vi "Tektronix TDS 3000 Series Dual channel Waveform Acquire.vi"() -> ()   [LabVIEW 2010]
doc: "DESCRIPTION:\nThis VI shows how to configure the Tektronix TDS 3xxx Series for a dual-channel waveform acquisition. It uses edge triggering to trigger the acquisition. \n\nINSTRUCTIONS:\n1. Pass a valid VISA session\n2. Enter a vertical offset, range and coupling for the specified channels.\n3. Enter the probe attenuation for the probe attached to the specified channel inputs.\n4. Enter the acquisition start time and desired time per record you want in the record.\n5. Enter the trigger level for the edge trigger.\n6. Run the VI.\n7. The acquired waveforms will be displayed in the graph.\n\nNOTES:\nNotice the order of the Tektronix tktd3k component VIs in the block diagram.\n\nThis VI sets the following controls on the block diagram:\n 20MHz Max Input Frequency.\n 1.0M Ohm Input Impedance.\n 500ns trigger holdoff.\n Edge trigger is DC coupled with a positive slope.\nTo change these controls, modify the associated block diagram constants."
uses:
  <instrlib>/Tektronix TDS 3000 Series/Tektronix TDS 3000 Series.lvlib
panel:
  in  "Acquisition Start Time (0.0 s)":dbl format="%.2p"
  in  "Trigger Source (Chan 1)":string(combo)="CH1"
  in  "Trigger Level (1.0 V)":dbl=1.0 format="%.2p"
  in  "Time Per Record (4.0e-3 s)":dbl=0.004 format="%.2p"
  in  "Vertical Offset (0.0 V)":dbl format="%.3p"
  in  "Vertical Range (10.0 V)":dbl=10.0 format="%.2p"
  in  "Probe Attenuation (1.0)":dbl=1.0 format="%.2f"
  in  "Vertical Coupling (DC)":i32(slide)=1
  in  "Channel Name (\"CH2\")":string(combo)="CH2"
  in  "Vertical Offset (0.0 V)":dbl format="%.3p"
  in  "Vertical Range (10.0 V)":dbl=10.0 format="%.2p"
  in  "Probe Attenuation (1.0)":dbl=1.0 format="%.2f"
  in  "Vertical Coupling (DC)":i32(slide)=1
  in  "Channel Name (\"CH1\")":string(combo)="CH1"
  out "Waveform Graph":T1(graph)
  in  "VISA resource name":refnum<visa-resource-name>="GPIB0::1::INSTR"
  # "© 2003-2006, National Instruments, Corporation.  All Rights Reserved."
  # "Horizontal Configuration"
  # "Triggering (Channel A)"
  # "For instructions,\nselect Show Context Help\nfrom the Help menu."
  # "Channel A Configuration"
  # "Channel B Configuration"
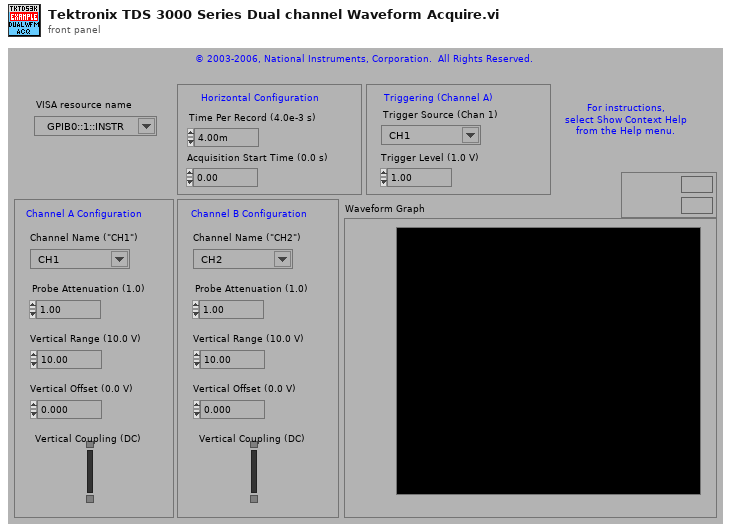
[diagram p1: front panel]
types:
  T1 = cluster{"initial x":dbl, "x increment":dbl, "waveform array":dbl[]}[]
  T2 = cluster{"Baud Rate (9600)":u32, "Flow Control (RTS/CTS)":u16, i32}
  T3 = cluster{"Initial X":dbl, "X Increment":dbl, "Waveform Array":dbl[]}
  T4 = cluster{"Initial X":dbl, "X Increment":dbl, "Waveform Array":dbl[]}[]
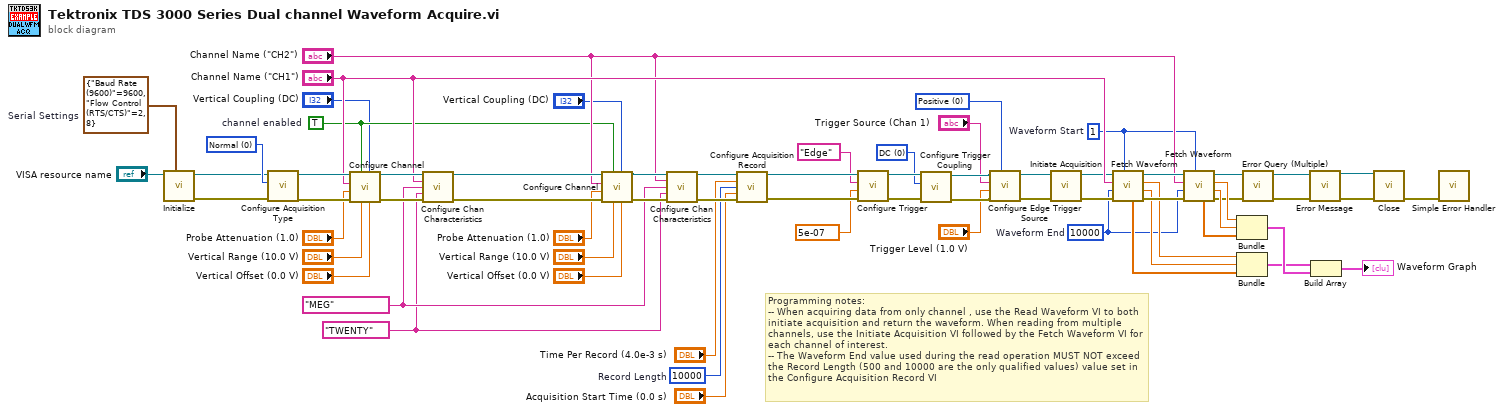
[diagram p0: block diagram]
diagram:
  w1 = "TWENTY" ("Max Input Frequency (20.0E+6 Hz)")
  w2 = 10000  # Waveform End
  w3 = 1  # Waveform Start
  w4 = 10000  # Record Length
  w17 = T2 {"Baud Rate (9600)"=9600, "Flow Control (RTS/CTS)"=2, 8}  # Serial Settings
  w53 = 0 items=["Normal", "Peak Detect", "Envelope", "Average"] ("Acquisition Type (0:Normal)")
  w46 = "MEG" ("Input Impedance (1.0 mega ohm)")
  w55 = u32 0 items=["DC", "High Frequency Reject", "Low Frequency Reject", "Noise Reject"] ("Trigger Coupling (DC)")
  w56 = 0 items=["Positive", "Negative"] ("Trigger Slope (Positive)")
  w32 = TRUE  # channel enabled
  # "Programming notes:\n-- When acquiring data from only channel , use the Read Waveform VI to both initiate acquisition and return the waveform. When reading from multiple channels, use the Initiate Acquisition VI followed by the Fetch Waveform VI for each channel of interest. \n-- The Waveform End value used during the read operation MUST NOT exceed the Record Length (500 and 10000 are the only qualified values) value set in the Configure Acquisition Record VI"
  n1 = call <instrlib>:"Initialize.vi"("Serial Settings"=w17, "VISA Resource Name"="VISA resource name") -> ("error out"=w19:errorcluster, "VISA Resource Name Out"=w18:refnum<visa-resource-name>)  [unwired: 8 in]
  n2 = call <instrlib>:"Configure Acquisition Type.vi"("error in (no error)"=w19, "Acquisition Type (0:Sample)"=w53, "VISA Resource Name"=w18) -> ("error out"=w67:errorcluster, "VISA Resource Name Out"=w65:refnum<visa-resource-name>)  [unwired: 7 in]
  n3 = call <instrlib>:"Configure Channel.vi"("Vertical Offset (0.0 V)"="Vertical Offset (0.0 V)", "Vertical Coupling (DC)"="Vertical Coupling (DC)", "Vertical Range (10.0 V)"="Vertical Range (10.0 V)", "Channel Enabled (True)"=w32, "error in (no error)"=w67, "Probe Attenuation (1.0)"="Probe Attenuation (1.0)", "Channel Name (\"CH1\")"="Channel Name (\"CH1\")", "VISA Resource Name"=w65) -> ("error out"=w66:errorcluster, "VISA Resource Name Out"=w64:refnum<visa-resource-name>)  [unwired: 2 in]
  n4 = call <instrlib>:"Configure Chan Characteristics.vi"("VISA Resource Name"=w64, "Channel Name (\"CH1\")"="Channel Name (\"CH1\")", "Input Impedance (1.0 mega ohm)"=w46, "Max Input Frequency (20.0E+6 Hz)"=w1, "error in (no error)"=w66) -> ("VISA Resource Name Out"=w52:refnum<visa-resource-name>, "error out"=w51:errorcluster)  [unwired: 9 in]
  n5 = call <instrlib>:"Configure Channel.vi"("Vertical Offset (0.0 V)"="Vertical Offset (0.0 V)", "Vertical Coupling (DC)"="Vertical Coupling (DC)", "Vertical Range (10.0 V)"="Vertical Range (10.0 V)", "Channel Enabled (True)"=w32, "error in (no error)"=w51, "Probe Attenuation (1.0)"="Probe Attenuation (1.0)", "Channel Name (\"CH1\")"="Channel Name (\"CH2\")", "VISA Resource Name"=w52) -> ("error out"=w50:errorcluster, "VISA Resource Name Out"=w49:refnum<visa-resource-name>)  [unwired: 2 in]
  n6 = call <instrlib>:"Configure Chan Characteristics.vi"("VISA Resource Name"=w49, "Channel Name (\"CH1\")"="Channel Name (\"CH2\")", "Input Impedance (1.0 mega ohm)"=w46, "Max Input Frequency (20.0E+6 Hz)"=w1, "error in (no error)"=w50) -> ("VISA Resource Name Out"=w48:refnum<visa-resource-name>, "error out"=w47:errorcluster)  [unwired: 9 in]
  n7 = call <instrlib>:"Configure Acquisition Record.vi"("VISA Resource Name"=w48, "Time Per Record (4.0e-3 s)"="Time Per Record (4.0e-3 s)", "Record Length (10000)"=w4, "Acquisition Start Time (0.0 s)"="Acquisition Start Time (0.0 s)", "error in (no error)"=w47) -> ("VISA Resource Name Out"=w63:refnum<visa-resource-name>, "error out"=w62:errorcluster)  [unwired: 9 in]
  n8 = call <instrlib>:"Configure Trigger.vi"("error in (no error)"=w62, "Trigger Holdoff (0.00 sec)"=5e-07 ("trigger holdoff (500ns)"), "Trigger Type (Edge)"="Edge", "VISA Resource Name"=w63) -> ("error out"=w58:errorcluster, "VISA Resource Name Out"=w60:refnum<visa-resource-name>)  [unwired: 6 in]
  n9 = call <instrlib>:"Configure Trigger Coupling.vi"("error in (no error)"=w58, "Trigger Coupling (DC)"=w55, "VISA Resource Name"=w60) -> ("error out"=w57:errorcluster, "VISA Resource Name Out"=w59:refnum<visa-resource-name>)  [unwired: 7 in]
  n10 = call <instrlib>:"Configure Edge Trigger Source.vi"("Trigger Slope (Positive)"=w56, "error in (no error)"=w57, "Trigger Level (0.0 V)"="Trigger Level (1.0 V)", "Trigger Source (Channel 1)"="Trigger Source (Chan 1)", "VISA Resource Name"=w59) -> ("error out"=w44:errorcluster, "VISA Resource Name Out"=w45:refnum<visa-resource-name>)  [unwired: 5 in]
  n11 = call <instrlib>:"Initiate Acquisition.vi"("error in (no error)"=w44, "VISA Resource Name"=w45) -> ("error out"=w8:errorcluster, "VISA Resource Name Out"=w7:refnum<visa-resource-name>)  [unwired: 8 in]
  n12 = call <instrlib>:"Fetch Waveform.vi"("Waveform Start (1)"=w3, "error in (no error)"=w8, "Waveform End (10000)"=w2, "Source (Channel 1)"="Channel Name (\"CH1\")", "VISA Resource Name"=w7) -> ("error out"=w43:errorcluster, "X Increment"=w38:dbl, "Initial X"=w39:dbl, "VISA Resource Name Out"=w42:refnum<visa-resource-name>, "Waveform Array"=w37:dbl[])  [unwired: 1 in, 1 out]
  n13 = call <instrlib>:"Fetch Waveform.vi"("Waveform Start (1)"=w3, "error in (no error)"=w43, "Waveform End (10000)"=w2, "Source (Channel 1)"="Channel Name (\"CH2\")", "VISA Resource Name"=w42) -> ("error out"=w10:errorcluster, "X Increment"=w35:dbl, "Initial X"=w34:dbl, "VISA Resource Name Out"=w11:refnum<visa-resource-name>, "Waveform Array"=w36:dbl[])  [unwired: 1 in, 1 out]
  n14 = Bundle("Initial X"=w34, "X Increment"=w35, "Waveform Array"=w36) -> (w21:T3)  [unwired: 1 in]
  n15 = Bundle("Initial X"=w39, "X Increment"=w38, "Waveform Array"=w37) -> (w20:T3)  [unwired: 1 in]
  n16 = call <instrlib>:"Error Query (Multiple).vi"("error in (no error)"=w10, "VISA Resource Name"=w11) -> ("error out"=w14:errorcluster, "VISA Resource Name Out"=w15:refnum<visa-resource-name>)  [unwired: 6 in, 2 out]
  n17 = call <instrlib>:"Error Message.vi"("VISA Resource Name"=w15, "error in (no error)"=w14) -> ("VISA Resource Name Out"=w13:refnum<visa-resource-name>, "error out"=w12:errorcluster)  [unwired: 9 in, 3 out]
  n18 = Build Array(w20, w21) -> (→"Waveform Graph":T4)
  n19 = call <instrlib>:"Close.vi"("error in (no error)"=w12, "VISA Resource Name"=w13) -> ("error out"=w9:errorcluster)  [unwired: 9 in]
  n20 = call <vilib>:"Simple Error Handler.vi"("error in (no error)"=w9) -> ()  [unwired: 4 in, 5 out]
